vi "Error Query (Multiple).vi"(0 "VISA resource name":refnum<visa-resource-name>, 11 "error in (no error)":errorcluster) -> (4 "VISA resource name out":refnum<visa-resource-name>, 8 "Error":i32[](array[numeric]), 10 "Error Message":string, 15 "error out":errorcluster)   [LabVIEW 2013, in "Fluke 5XXX Series Multicalibrators.lvlib"]
doc: "This VI reads the error queue from the instrument. It expects to see errors in SCPI format (#,\"error message\"). It continues to read from the error queue until it reads a 0, \"No error\". If the instrument does not support an error query, a warning is returned."
uses:
  Fluke 5XXX Series Multicalibrators.lvlib
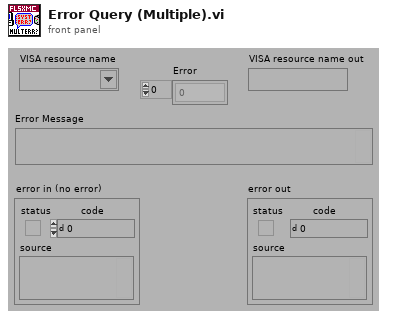
[diagram p1: front panel]
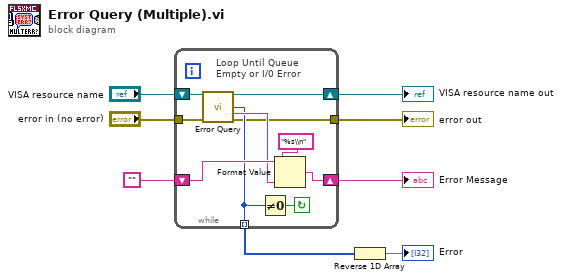
[diagram p0: block diagram]
diagram:
  n1 = while {
    tunnel: "error in (no error)" -> [w9]
    tunnel: [w12] -> w3 mode=indexing
    tunnel: [w10] -> w1
    shift-left: "VISA resource name" -> [w11]
    shift-right: [w18] -> w7
    shift-left: "" -> [w15]
    shift-right: [w17] -> w6
    stop <- w13 continue-if-true
    # "Loop Until Queue Empty or I/0 Error"
    n2 = call "Error Query.vi"("VISA resource name"=w11, "error in (no error)"=w9) -> ("VISA resource name out"=w18:refnum<visa-resource-name>, "Error Code"=w12:i32, "Error Message"=w14:string, "error out"=w10:errorcluster)  [unwired: 10 in]
    n3 = Not Equal To 0?(x=w12) -> (x != 0?=w13:bool)
    n4 = Format Value(string ("")=w15, format string="%s\\n", value (0)=w14) -> (output string=w17:string)
  }
  "Error Message" <- w6
  "error out" <- w1
  "VISA resource name out" <- w7
  n5 = Reverse 1D Array(array=w3) -> (reversed array=→"Error":i32[])
